vi "Initialize.vi"(8 "error in":errorcluster) -> (0 "error out":errorcluster, 3 "ARINC 429 (32-bit word)":refnum<class "32-bit Word.lvclass">)   [LabVIEW 2020, in "32-bit Word.lvclass"]
uses:
  32-bit Word.lvclass
  C:/Git/Ballard-ARINC429-custom-device/ARINC429/ARINC 429.lvclass
  ARINC 429.lvclass/ARINC 429.ctl
  32-bit Word.lvclass/32-bit Word.ctl
  Write Label Start Index.vi
  Write Label Size.vi
  Write Data Start Index.vi
  Write Data Size.vi
  Write Parity Start Index.vi
  Write Parity.vi
  Write Label Value.vi
  Write 32-Bit Word.vi
  Write SDI Start Index.vi
  Write SDI Size.vi
  Write SSM Start Index.vi
  Write SSM Size.vi
  Write SDI Value.vi
  Write SSM Value.vi
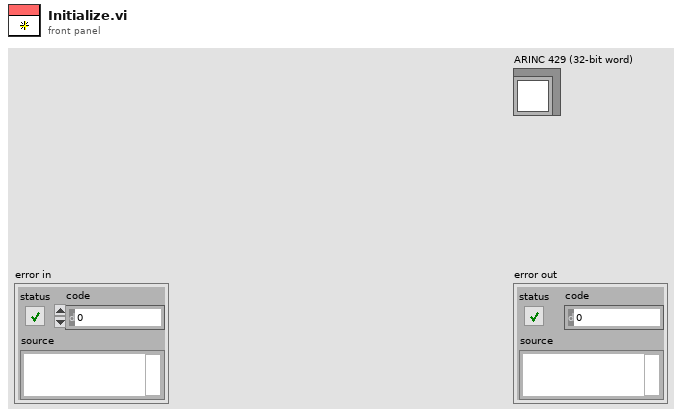
[diagram p1: front panel]
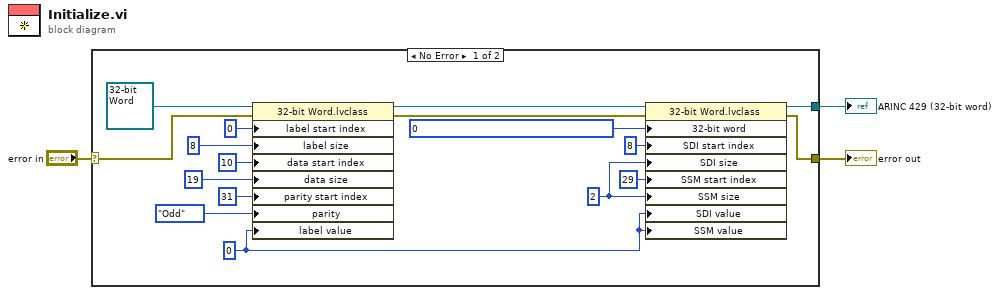
[diagram p0: block diagram]
diagram:
  n1 = case shown="No Error" "error in" {
    selector: "error in" -> [w18 w21]
    tunnel: [w7 w21] -> w2
    tunnel: [w6 _] -> w1
    frame No Error {
      w5 = u8 0 ("label value")
      w8 = 2 ("SDI size")
      n2 = property on="Property Node" class="32-bit Word.lvclass"(reference=refnum<class "32-bit Word.lvclass"> refnum ("32-bit Word.lvclass"), error in=w18, "label start index"=0, "label size"=8, "data start index"=10, "data size"=19, "parity start index"=31, "parity"=enum16{"Even", "Odd"}."Odd", "label value"=w5) -> (reference out=w19:refnum<class "32-bit Word.lvclass">, error out=w11:errorcluster)
      n3 = property on="Property Node" class="32-bit Word.lvclass"(reference=w19, error in=w11, "32-bit word"=u32 0, "SDI start index"=8, "SDI size"=w8, "SSM start index"=29, "SSM size"=w8, "SDI value"=w5, "SSM value"=w5) -> (reference out=w6:refnum<class "32-bit Word.lvclass">, error out=w7:errorcluster)
    }
    frame Error {
    }
  }
  "error out" <- w2
  "ARINC 429 (32-bit word)" <- w1
